vi "Autonomous Independent.vi"   [LabVIEW 2018]
doc: "This VI is called when autonomous begins, and will automatically be terminated when autonomous ends. You can carry out timed or sensor driven robot movement independently without needing to return to the caller."
uses:
  <vilib>/Rock Robotics/Network Tables/NT Write Number.vi
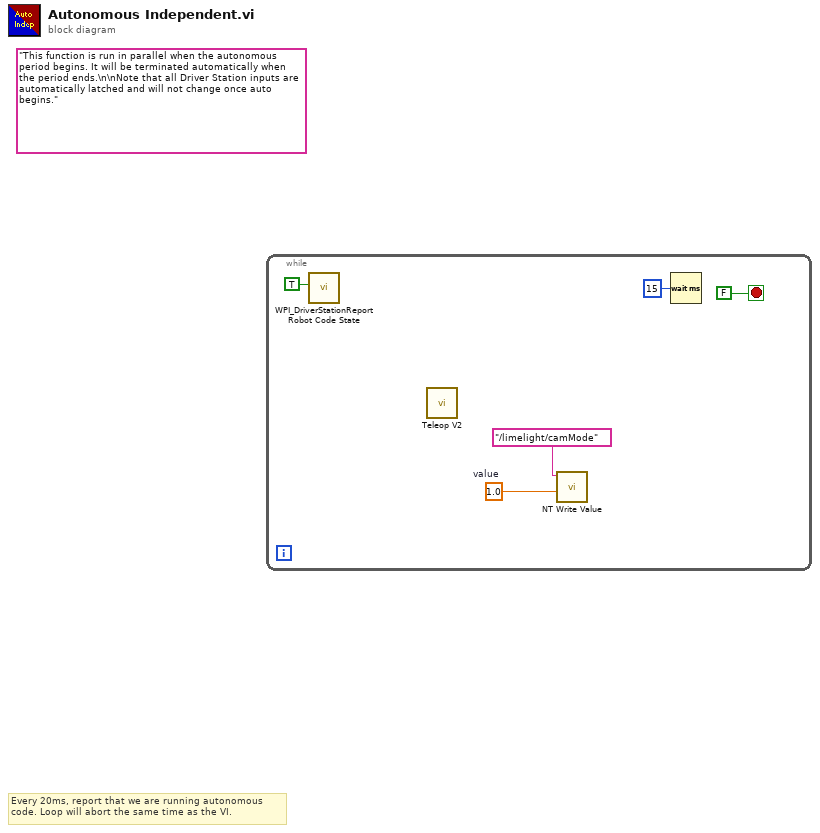
[diagram p0: block diagram]
diagram:
  (unwired) "This function is run in parallel when the autonomous period begins. It will be terminated automatically when the period ends.\n\nNote that all Driver Station inputs are automatically latched and will not change once auto begins."
  # "Every 20ms, report that we are running autonomous\ncode. Loop will abort the same time as the VI."
  n1 = while {
    stop <- FALSE stop-if-true
    w1 = 1.0  # value
    n2 = call <vilib>:"WPI_DriverStationReport Robot Code State.vi"("Autonomous"=TRUE) -> ()  [unwired: 10 in, 1 out]
    n3 = call "Teleop V2.vi"() -> ()  [unwired: 12 in]
    n4 = call-poly <vilib>:"NT Write Value.vi"("Numeric"=w1, "Name"="/limelight/camMode") -> ()  [unwired: 9 in, 1 out]
    n5 = Wait (ms)(milliseconds to wait=u32 15) -> ()  [unwired: 1 out]
  }
